vi "GA Ln XY.vi"(0 "nCrdNum":i16, 1 "synAcc":dbl, 2 "FifoIndex":i16, 5 "x":i32, 7 "y":i32, 9 "synVel":dbl, 11 "error in (no error)":errorcluster caption="错误输入（无错误）", 12 "velEnd":dbl, 13 "segNum":i32) -> (4 "function return":i32, 15 "error out":errorcluster caption="错误输出")   [LabVIEW 2015, in "GAS.lvlib"]
doc: "extern \"C\" __declspec(dllimport) int GA_LnXY(short nCrdNum,long x,long y,double synVel,double synAcc,double velEnd=0,short FifoIndex=0,long segNum = 0);"
uses:
  <userlib>/BP_GAS/GAS.lvlib
  <userlib>/BP_GAS/GAS.dll
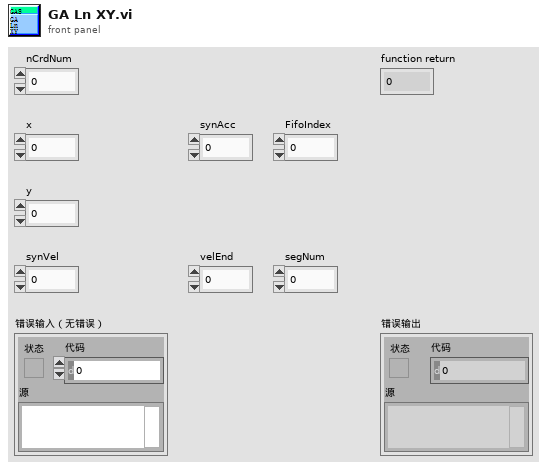
[diagram p1: front panel]
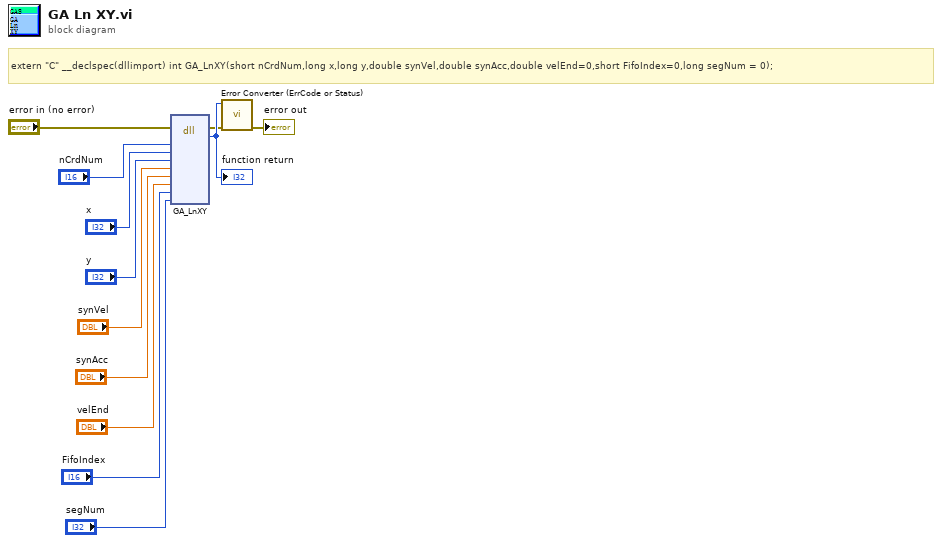
[diagram p0: block diagram]
diagram:
  # "extern \"C\" __declspec(dllimport) int GA_LnXY(short nCrdNum,long x,long y,double synVel,double synAcc,double velEnd=0,short FifoIndex=0,long segNum = 0);"
  n1 = dll-call lib="E:/Program Files (x86)/National Instruments/LabVIEW 2015/user.lib/BP_GAS/GAS.*" fn="GA_LnXY"(error in="error in (no error)", "nCrdNum"="nCrdNum", "x"="x", "y"="y", "synVel"="synVel", "synAcc"="synAcc", "velEnd"="velEnd", "FifoIndex"="FifoIndex", "segNum"="segNum") -> (error out=w2:errorcluster, w12:i32)  [unwired: 10 in, 1 out]
  "function return" <- w12
  n2 = call "Error Converter (ErrCode or Status).vi"("error in (no error)"=w2, "error code"=w12) -> ("error out"=→"error out":errorcluster)  [unwired: 9 in]
